vi "UICreateConfig.vi"() -> ()   [LabVIEW 2014]
uses:
  <vilib>/Utility/config.llb/Write Key (Double).vi
  <vilib>/Utility/config.llb/Write Key (Path).vi
  <vilib>/Utility/config.llb/Read Key (Path).vi
  <vilib>/Utility/config.llb/NI_LVConfig.lvlib
panel:
  in  "PusherPositionsArray":dbl[](array[numeric])
  in  "LiftInputArray":dbl[](array[numeric])
  in  "PositionArrayPath 2":path
  in  "PusherThreshold":dbl format="%#_13g"
  in  "PusherPositionRequested":dbl format="%#_13g"
  in  "LiftInputArrayPath":path
  in  "LiftRequestedHeight":dbl format="%#_13g"
  in  "LiftThreshold":dbl format="%#_13g"
  in  "LiftMotorSpeedUp":dbl format="%#_13g"
  in  "LiftMotorSpeedDown":dbl format="%#_13g"
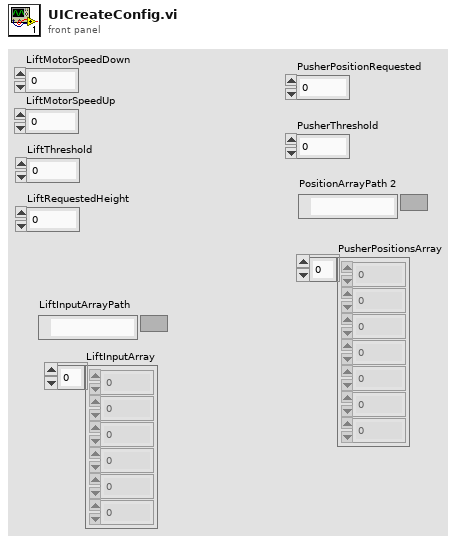
[diagram p1: front panel]
types:
  T1 = enum16{"open", "replace", "create", "open or create", "replace or create", "replace or create with confirmation"}
  T2 = typedef "NI_LVConfig.lvlib/Config Data RefNum.ctl" = refnum<k1>
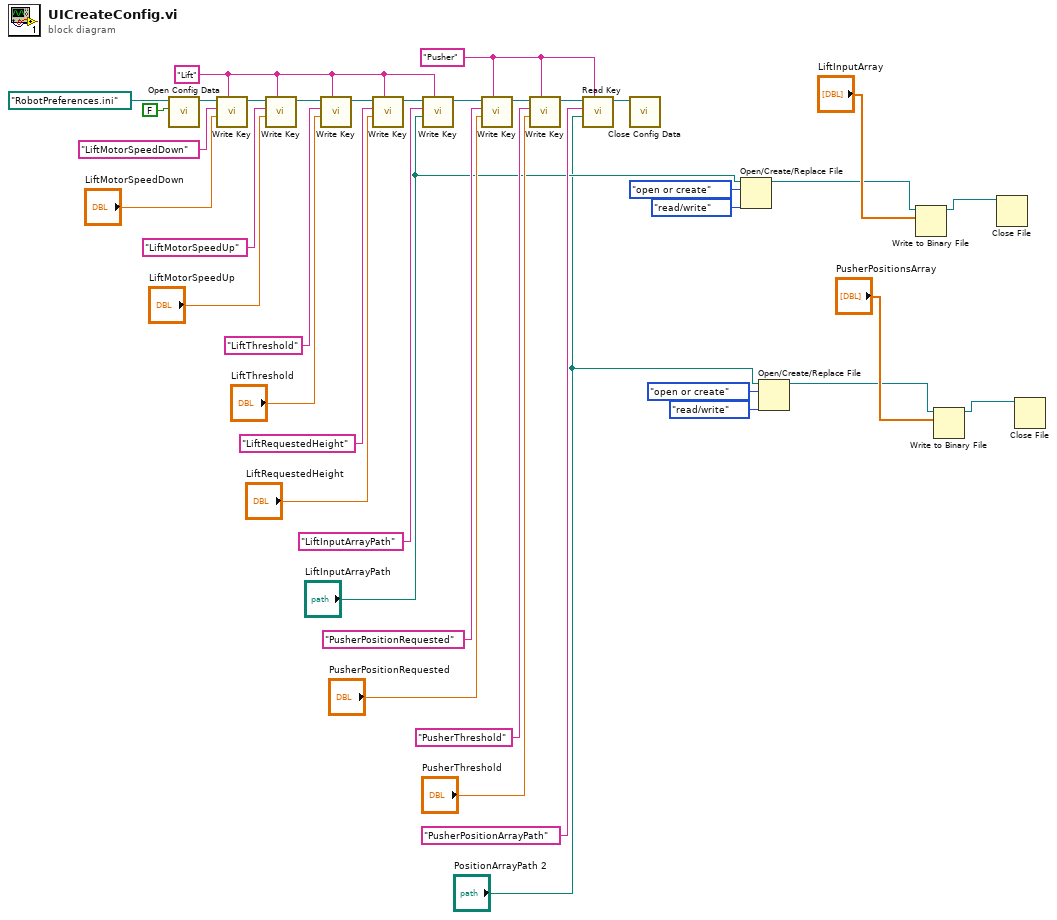
[diagram p0: block diagram]
diagram:
  w24 = "Pusher" ("section")
  w21 = "Lift" ("section")
  n1 = call <vilib>:"Open Config Data.vi"("create file if necessary (T)"=FALSE, "configuration file path"=path "RobotPreferences.ini") -> ("refnum"=w37:T2)  [unwired: 7 in, 2 out]
  n2 = call-poly <vilib>:"Write Key.vi"("section"=w21, "value"="LiftMotorSpeedDown", "key"="LiftMotorSpeedDown", "refnum"=w37) -> ("refnum out"=w20:T2)  [unwired: 5 in, 2 out]
  n3 = call-poly <vilib>:"Write Key.vi"("section"=w21, "value"="LiftMotorSpeedUp", "key"="LiftMotorSpeedUp", "refnum"=w20) -> ("refnum out"=w34:T2)  [unwired: 5 in, 2 out]
  n4 = call-poly <vilib>:"Write Key.vi"("section"=w21, "value"="LiftThreshold", "key"="LiftThreshold", "refnum"=w34) -> ("refnum out"=w32:T2)  [unwired: 5 in, 2 out]
  n5 = call-poly <vilib>:"Write Key.vi"("section"=w21, "value"="LiftRequestedHeight", "key"="LiftRequestedHeight", "refnum"=w32) -> ("refnum out"=w27:T2)  [unwired: 5 in, 2 out]
  n6 = call-poly <vilib>:"Write Key.vi"("section"=w21, "value"="LiftInputArrayPath", "key"="LiftInputArrayPath", "refnum"=w27) -> ("refnum out"=w15:T2)  [unwired: 5 in, 2 out]
  n7 = call-poly <vilib>:"Write Key.vi"("section"=w24, "value"="PusherPositionRequested", "key"="PusherPositionRequested", "refnum"=w15) -> ("refnum out"=w29:T2)  [unwired: 5 in, 2 out]
  n8 = call-poly <vilib>:"Write Key.vi"("section"=w24, "value"="PusherThreshold", "key"="PusherThreshold", "refnum"=w29) -> ("refnum out"=w25:T2)  [unwired: 5 in, 2 out]
  n9 = call-poly <vilib>:"Read Key.vi"("section"=w24, "default value"="PositionArrayPath 2", "key"="PusherPositionArrayPath", "refnum"=w25) -> ("refnum out"=w22:T2)  [unwired: 4 in, 3 out]
  n10 = call <vilib>:"Close Config Data.vi"("refnum"=w22) -> ()  [unwired: 9 in, 2 out]
  n11 = Open/Create/Replace File(file path (use dialog)="LiftInputArrayPath", operation (0:open)=T1."open or create", access (0:read/write)=enum16{"read/write", "read-only", "write-only"}."read/write") -> (refnum out=w8:refnum<file>)  [unwired: 3 in, 2 out]
  n12 = Open/Create/Replace File(file path (use dialog)="PositionArrayPath 2", operation (0:open)=T1."open or create", access (0:read/write)=enum16{"read/write", "read-only", "write-only"}."read/write") -> (refnum out=w3:refnum<file>)  [unwired: 3 in, 2 out]
  n13 = Write to Binary File(file (use dialog)=w8, data="LiftInputArray") -> (refnum out=w7:refnum<file>)  [unwired: 4 in, 2 out]
  n14 = Write to Binary File(file (use dialog)=w3, data="PusherPositionsArray") -> (refnum out=w2:refnum<file>)  [unwired: 4 in, 2 out]
  n15 = Close File(refnum=w7) -> ()  [unwired: 1 in, 2 out]
  n16 = Close File(refnum=w2) -> ()  [unwired: 1 in, 2 out]
